vi "LockinDAQ.Configure Sweep.vi"(8 "error in (no error)":errorcluster, 11 "LockinDAQ in":refnum<class "LockinDAQ.lvclass">) -> (0 "error out":errorcluster, 3 "LockinDAQ out":refnum<class "LockinDAQ.lvclass">)   [LabVIEW 2016, in "LockinDAQ.lvclass"]
uses:
  LockinDAQ.lvclass
  Typedefs/Function-enum.ctl
  LockinDAQ.lvclass/LockinDAQ.ctl
panel:
  out "Frequency (Hz)":dbl
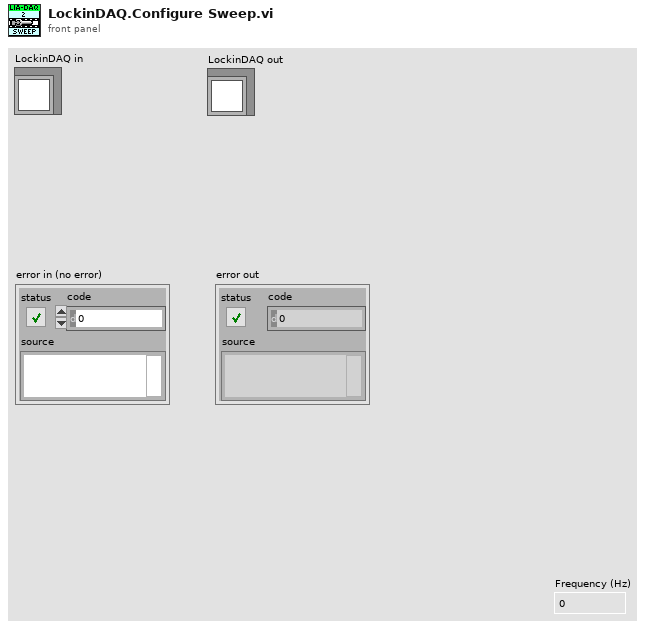
[diagram p1: front panel]
types:
  T1 = typedef "LockinDAQ.lvclass/Function-enum.ctl" = enum16{"Sine", "Triangle", "Square", "Sawtooth"}
  T2 = typedef "LockinDAQ.lvclass/AO-cluster.ctl" = cluster{"Ch":i32[], "Amp (V)":dbl[], "DC (V)":dbl[], "f (Hz)":dbl[], "Phase (°)":dbl[], "Function":T1[], "Sweep?":bool[]}
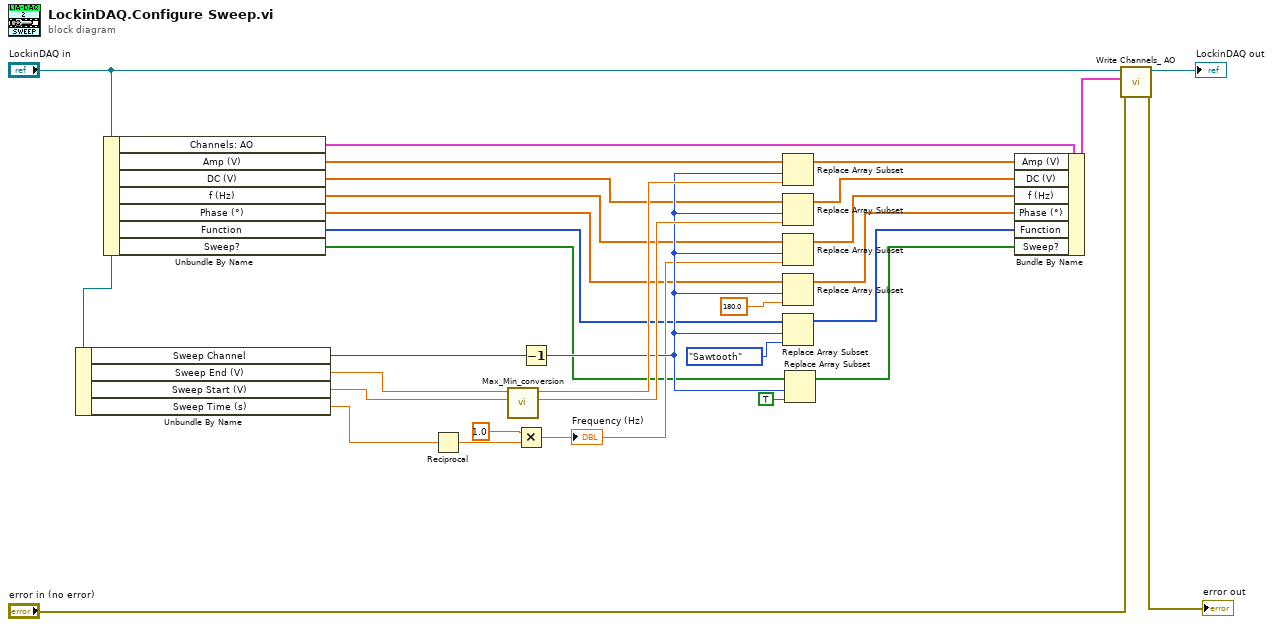
[diagram p0: block diagram]
diagram:
  n1 = Unbundle By Name("LockinDAQ in") -> ("Sweep Channel"=w4:i32, "Sweep End (V)"=w5:dbl, "Sweep Start (V)"=w6:dbl, "Sweep Time (s)"=w1:dbl)
  n2 = Unbundle By Name("LockinDAQ in") -> ("Channels: AO"=w3:T2, "Amp (V)"=w18:dbl[], "DC (V)"=w17:dbl[], "f (Hz)"=w16:dbl[], "Phase (°)"=w15:dbl[], "Function"=w14:T1[], "Sweep?"=w13:bool[])
  n3 = Reciprocal(x=w1) -> (1/x=w26:dbl)
  n4 = call <userlib>:"Max_Min_conversion.vi"("Min"=w6, "Max"=w5) -> ("offset"=w24:dbl, "Amplitude"=w25:dbl)  [unwired: 8 in]
  n5 = Multiply(x=1.0, y=w26) -> (x*y=w20:dbl)
  "Frequency (Hz)" <- w20
  n6 = Decrement(x=w4) -> (x-1=w21:i32)
  n7 = Replace Array Subset(array=w18, new element=w25, index=w21) -> (w12:dbl[])
  n8 = Replace Array Subset(array=w17, new element=w24, index=w21) -> (w11:dbl[])
  n9 = Replace Array Subset(array=w16, new element=w20, index=w21) -> (w10:dbl[])
  n10 = Replace Array Subset(array=w15, new element=180.0 ("new element/subarray"), index=w21) -> (w9:dbl[])
  n11 = Replace Array Subset(array=w14, new element=Function-enum."Sawtooth" ("new element/subarray"), index=w21) -> (w8:T1[])
  n12 = Replace Array Subset(array=w13, new element=TRUE ("new element/subarray"), index=w21) -> (w7:bool[])
  n13 = Bundle By Name(cluster=w3, "Amp (V)"=w12, "DC (V)"=w11, "f (Hz)"=w10, "Phase (°)"=w9, "Function"=w8, "Sweep?"=w7) -> (w28:T2)
  n14 = call "Write Channels_ AO.vi"("error in (no error)"="error in (no error)", "Channels: AO"=w28, "LockinDAQ"="LockinDAQ in") -> ("error out"=→"error out":errorcluster, "LockinDAQ out"=→"LockinDAQ out":refnum<class "LockinDAQ.lvclass">)  [unwired: 7 in]
